vi "Set Global CSM Filter.vi"(10 "Group:CSM":string[](array[string]), 11 "GlobalLogFilter in":refnum<class "LogFilter.lvclass">) -> (3 "GlobalLogFilter out":refnum<class "LogFilter.lvclass">)   [LabVIEW 2020, in "Communicable State Machine.lvlib" / "LogFilter.lvclass"]
uses:
  LogFilter.lvclass
  LogFilter.lvclass/LogFilter.ctl
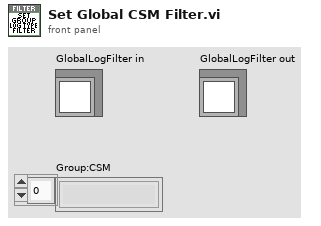
[diagram p1: front panel]
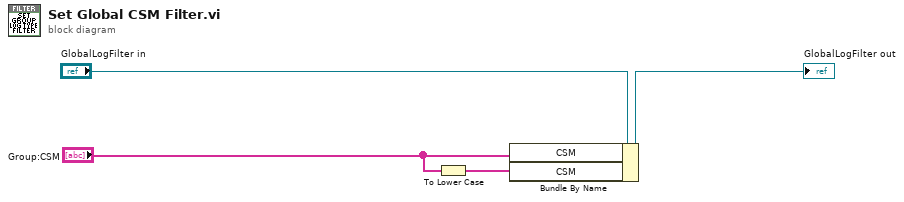
[diagram p0: block diagram]
diagram:
  n1 = To Lower Case(string="Group:CSM") -> (all lower case string=w1:string[])
  n2 = Bundle By Name(cluster="GlobalLogFilter in", "CSM"="Group:CSM", "CSM"=w1) -> (→"GlobalLogFilter out":refnum<class "LogFilter.lvclass">)
